vi "Read Info from File.vi"(8 "error in (no error)":errorcluster, 11 "LabVIEW Library File in":refnum<class "LabVIEW Library File.lvclass">) -> (0 "error out":errorcluster, 3 "LabVIEW Library File out":refnum<class "LabVIEW Library File.lvclass">)   [LabVIEW 2020, in "Save for Previous Version.lvlib" / "LabVIEW Library File.lvclass"]
uses:
  LabVIEW Library File.lvclass
  \\Mac\Home/JKI/GitHub/vipm-io/a-version-explorer-for-labview/experiments/save-for-previous-version/source/File/File.lvclass/File.lvclass
  \\Mac\Home/JKI/GitHub/vipm-io/a-version-explorer-for-labview/experiments/save-for-previous-version/source/LabVIEW File/LabVIEW File.lvclass
  File/File.lvclass/File.lvclass/File.ctl
  LabVIEW File/LabVIEW File.lvclass/LabVIEW File.ctl
  File/File.lvclass/Read Path.vi
  LabVIEW File/Write Version String.vi
  LabVIEW File/Write Version Number.vi
  LabVIEW File/LabVIEW File.lvclass
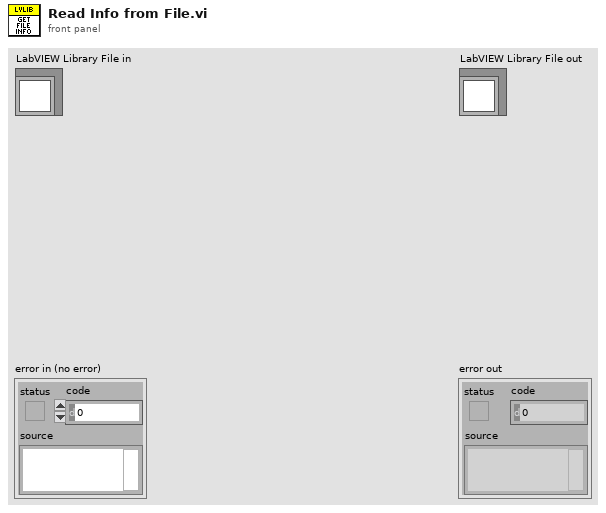
[diagram p1: front panel]
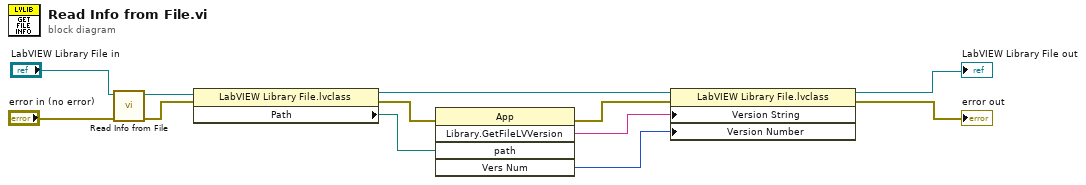
[diagram p0: block diagram]
diagram:
  n1 = call-parent "Read Info from File.vi"("error in (no error)"="error in (no error)", "LabVIEW File in"="LabVIEW Library File in") -> ("error out"=w3:errorcluster, "LabVIEW File out"=w4:refnum<class "LabVIEW Library File.lvclass">)  [unwired: 8 in]
  n2 = property class="LabVIEW Library File.lvclass"(reference=w4, error in=w3) -> (reference out=w8:refnum<class "LabVIEW Library File.lvclass">, error out=w6:errorcluster, "Path"=w7:path)
  n3 = invoke class="App" method="Library.GetFileLVVersion"(error in=w6, "path"=w7) -> (error out=w5:errorcluster, "Library.GetFileLVVersion"=w10:string, "Vers Num"=w9:u32)  [unwired: 3 in, 2 out]
  n4 = property class="LabVIEW Library File.lvclass"(reference=w8, error in=w5, "Version String"=w10, "Version Number"=w9) -> (reference out=→"LabVIEW Library File out":refnum<class "LabVIEW Library File.lvclass">, error out=→"error out":errorcluster)
